vi "OSC_exp_display.vi"() -> ()   [LabVIEW 2011]
doc: "Demonstrates how to set up an oscilloscope automatically. You can configure this VI to acquire a waveform from a single channel by following the following steps:\n\n1. Specify a valid VISA resource to use. \n2. Specify a channel. \n3. Specify a time-out value for reading a waveform.\n4. Run this VI. The <B>Waveform Graph</B> displays the waveform you acquire."
uses:
  global.vi
  <vilib>/measure/maspectr.llb/FFT Power Spectrum and PSD for 1 Chan.vi
  <instrlib>/Tektronix 7000 Series/Tektronix 7000 Series.lvlib
  <vilib>/measure/NI_MAPro.lvlib
panel:
  out "bg FD signal":cluster{"f0":dbl, "df":dbl, "magnitude":dbl[]}(graph)
  out "mol FD signal":cluster{"f0":dbl, "df":dbl, "magnitude":dbl[]}(graph)
  out "current ave corre FD":cluster{"f0":dbl, "df":dbl, "magnitude":dbl[]}(graph)
  out "current meas corre FD":cluster{"f0":dbl, "df":dbl, "magnitude":dbl[]}(graph)
  in  "stop meas":bool
  out "current average":i32
  out "current ave corre TD":dbl[](graph)
  in  "#averages":i32
  in  "Exit":bool
  in  "start":bool
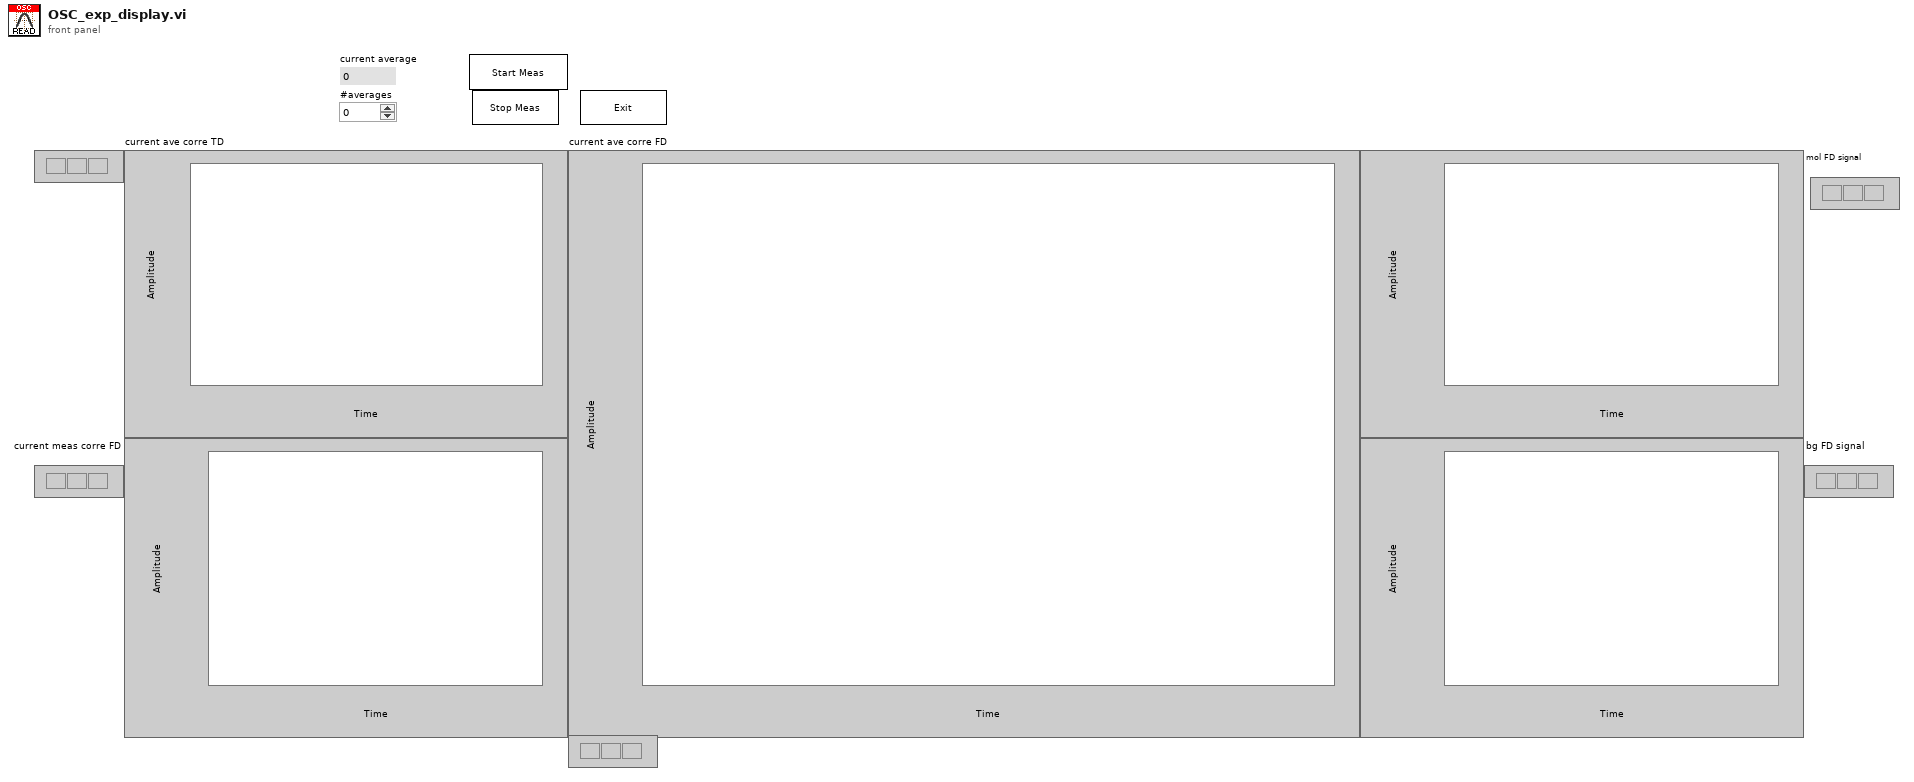
[diagram p1: front panel]
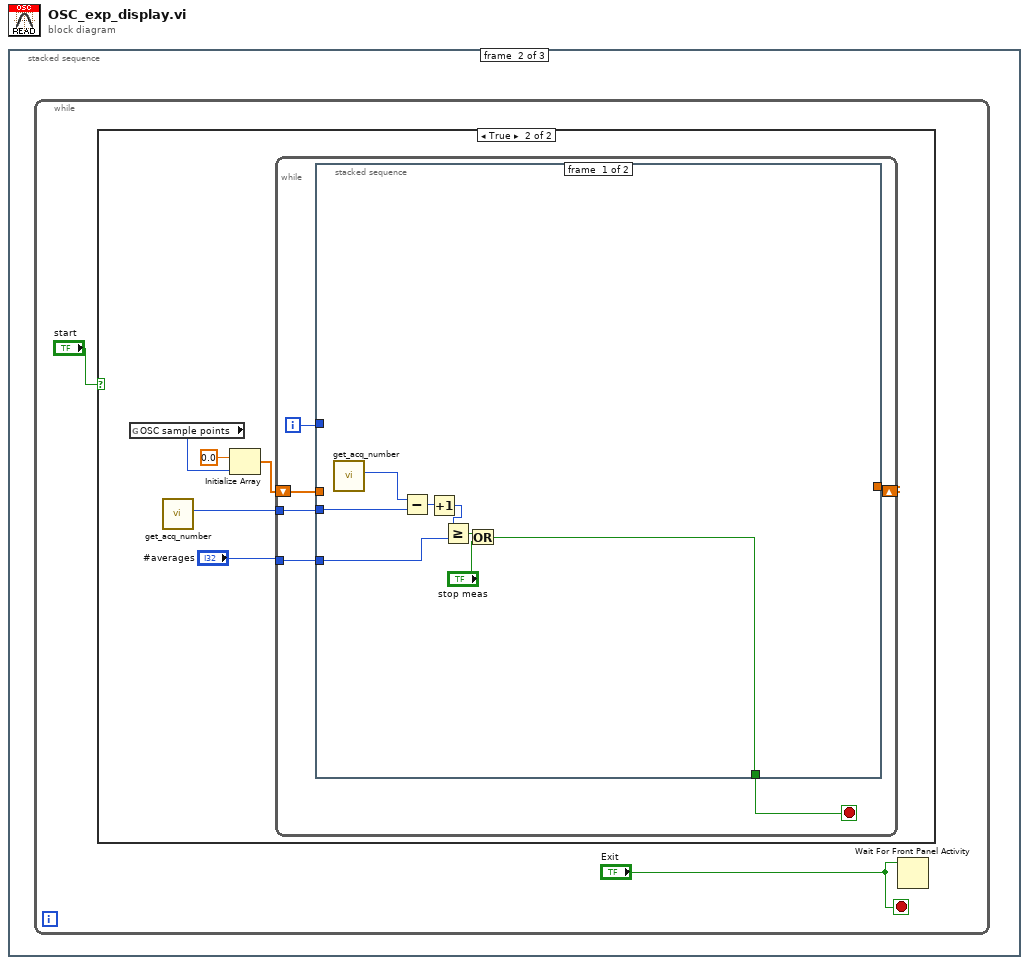
[diagram p0: block diagram]
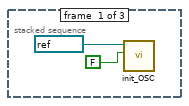
[diagram p2: hidden frame]
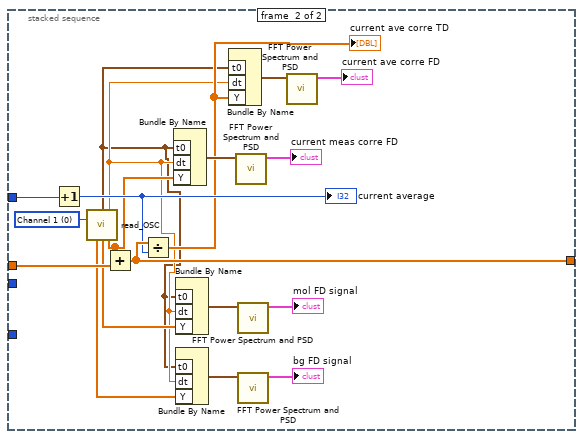
[diagram p4: hidden frame]
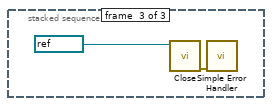
[diagram p5: hidden frame]
diagram:
  n1 = stacked-sequence {
    frame #0 {
      n2 = call "init_OSC.vi"("reset (f)"=FALSE, "VISA resource name"=refnum<visa-resource-name> "OSC" ("OSC")) -> ()  [unwired: 8 in, 2 out]
    }
    frame #1 {
      n3 = while {
        stop <- "Exit" stop-if-true
        n4 = case shown="True" "start" {
          frame False {
          }
          frame True {
            n5 = global read "global.vi" "OSC sample points"() -> (w7:i32)
            n6 = call "get_acq_number.vi"() -> ("# of meas cycles"=w5:i32)  [unwired: 8 in, 3 out]
            n7 = Initialize Array(0.0 ("element"), w7) -> (w8:dbl[])
            n8 = while {
              shift-right: [w14] -> _
              shift-left: w8 -> [w15]
              tunnel: "#averages" -> [w11]
              tunnel: w5 -> [w12]
              i -> [w13]
              stop <- w10 stop-if-true
              n9 = stacked-sequence {
                tunnel: w15 -> [_ w42]
                tunnel: [_ w41] -> w14
                tunnel: w13 -> [_ w40]
                tunnel: w12 -> [w20 _]
                tunnel: w11 -> [w19 _]
                tunnel: [w18 _] -> w10
                frame #0 {
                  n10 = call "get_acq_number.vi"() -> ("# of meas cycles"=w22:i32)  [unwired: 8 in, 3 out]
                  n11 = Subtract(x=w22, y=w20) -> (x-y=w17:i32)
                  n12 = Increment(x=w17) -> (x+1=w16:i32)
                  n13 = Greater Or Equal?(x=w16, y=w19) -> (x >= y?=w21:bool)
                  n14 = Or(x=w21, y="stop meas") -> (x .or. y?=w18:bool)
                }
                frame #1 {
                  w35 = u16 0 items=["Channel 1", "Channel 2", "Channel 3", "Channel 4", "Math 1", "Math 2", "Math 3", "Math 4", "Reference 1", "Reference 2", "Reference 3", "Reference 4"] ("Channel (0: Channel 1)")
                  n15 = Increment(x=w40) -> (x+1=w39:i32)
                  "current average" <- w39
                  n16 = call "read_OSC.vi"("Channel (0: Channel 1)"=w35) -> ("t0"=w24:timestamp, "dt"=w25:dbl, "ave. background TD signal"=w26:dbl[], "ave. molecularTD signal"=w27:dbl[], "cor. ave. TD signal"=w38:dbl[])  [unwired: 7 in, 3 out]
                  n17 = Add(x=w38, y=w42) -> (x+y=w41:dbl[])
                  n18 = Divide(x=w41, y=w39) -> (x/y=w33:dbl[])
                  "current ave corre TD" <- w33
                  n19 = Bundle By Name("t0"=w24, "dt"=w25, "Y"=w38) -> (w37:waveform(dbl))  [unwired: 1 in]
                  n20 = Bundle By Name("t0"=w24, "dt"=w25, "Y"=w27) -> (w31:waveform(dbl))  [unwired: 1 in]
                  n21 = Bundle By Name("t0"=w24, "dt"=w25, "Y"=w26) -> (w29:waveform(dbl))  [unwired: 1 in]
                  n22 = Bundle By Name("t0"=w24, "dt"=w25, "Y"=w33) -> (w32:waveform(dbl))  [unwired: 1 in]
                  n23 = call-poly <vilib>:"FFT Power Spectrum and PSD.vi"("time signal"=w37) -> ("Power Spectrum / PSD"=→"current meas corre FD":cluster{"f0":dbl, "df":dbl, "magnitude":dbl[]})  [unwired: 7 in, 3 out]
                  n24 = call-poly <vilib>:"FFT Power Spectrum and PSD.vi"("time signal"=w31) -> ("Power Spectrum / PSD"=→"mol FD signal":cluster{"f0":dbl, "df":dbl, "magnitude":dbl[]})  [unwired: 7 in, 3 out]
                  n25 = call-poly <vilib>:"FFT Power Spectrum and PSD.vi"("time signal"=w29) -> ("Power Spectrum / PSD"=→"bg FD signal":cluster{"f0":dbl, "df":dbl, "magnitude":dbl[]})  [unwired: 7 in, 3 out]
                  n26 = call-poly <vilib>:"FFT Power Spectrum and PSD.vi"("time signal"=w32) -> ("Power Spectrum / PSD"=→"current ave corre FD":cluster{"f0":dbl, "df":dbl, "magnitude":dbl[]})  [unwired: 7 in, 3 out]
                }
              }
            }
          }
        }
        n27 = Wait For Front Panel Activity(3:"Exit") -> ()  [unwired: 2 in, 1 out]
      }
    }
    frame #2 {
      n28 = call <instrlib>:"Close.vi"("VISA resource name"=refnum<visa-resource-name> "OSC" ("OSC")) -> ("error out"=w43:errorcluster)  [unwired: 10 in]
      n29 = call <vilib>:"Simple Error Handler.vi"("error in (no error)"=w43) -> ()  [unwired: 4 in, 5 out]
    }
  }
